vi "SPI_ReadBytes.vi"(5 "Device":i32, 6 "Length":i32, 7 "Bus":i32=1, 8 "error in":errorcluster) -> (0 "error out":errorcluster, 4 "Bytes":u8[](array[numeric]) format="%.0x")   [LabVIEW 2014, in "GPIO.lvlib"]
doc: "Read bytes from the specified device"
uses:
  GPIO.lvlib
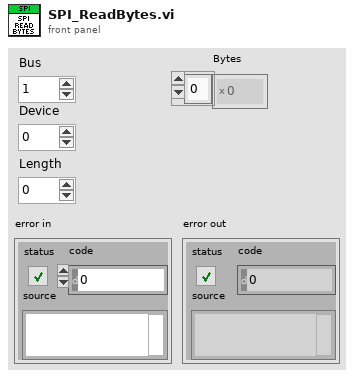
[diagram p1: front panel]
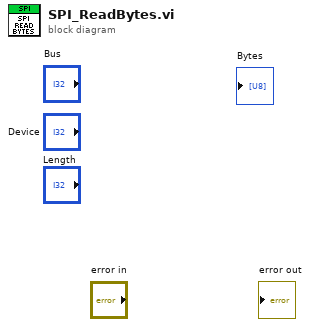
[diagram p0: block diagram]
diagram:
